vi "USB Flash Drive Action.vi"(8 "error in (no error)":errorcluster, 9 "number in file name":u8, 10 "action":u16(ring)=2 items=["load"=2, "format"=3, "delete"=4], 11 "VGC in":refnum<class "PL Inficon VGC.lvclass">) -> (0 "error out":errorcluster, 2 "state":u16(ring) items=["loaded", "loading", "load", "format", "delete"], 3 "VGC out":refnum<class "PL Inficon VGC.lvclass">)   [LabVIEW 2015, in "PL Inficon VGC.lvclass"]
doc: "Loads parameters from USB."
uses:
  PL Inficon VGC.lvclass
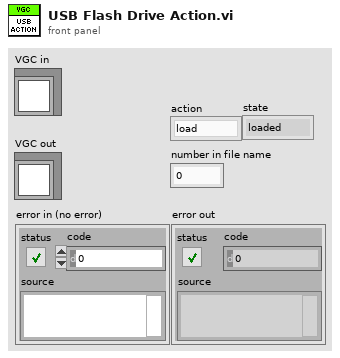
[diagram p1: front panel]
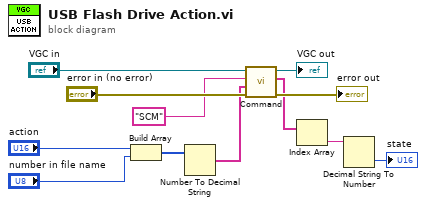
[diagram p0: block diagram]
diagram:
  n1 = Build Array("action", "number in file name") -> (w5:u16[])
  n2 = Number To Decimal String(number=w5) -> (decimal integer string=w6:string[])  [unwired: 1 in]
  n3 = call "Command.vi"("error in (no error)"="error in (no error)", "parameters"=w6, "command"="SCM", "VGC in"="VGC in") -> ("error out"=→"error out":errorcluster, "response data"=w3:string[], "VGC out"=→"VGC out":refnum<class "PL Inficon VGC.lvclass">)  [unwired: 5 in]
  n4 = Index Array(array=w3) -> (element=w2:string)  [unwired: 1 in]
  n5 = Decimal String To Number(string=w2) -> (number=→"state":i32)  [unwired: 2 in, 1 out]
